vi "Create ActorRef Queue.vi"(11 "Core In":refnum<class "Core.lvclass">) -> (0 "Error Out":errorcluster, 3 "Core Out":refnum<class "Core.lvclass">)   [LabVIEW 2019, in "Core.lvlib" / "Core.lvclass"]
uses:
  Core.lvclass
  C:/Projekty/_Wewnetrzne/PC_ActorFramework/07_Program/LABVIEW/02_Source/Modules/ModuleAbstract/ModuleAbstract.lvclass
  Containers/ActorRefContainer/ActorRefContainer.lvclass
  Containers/ActorRefContainer/ActorRefContainer.lvclass/ActorRefContainer.ctl
  Core.lvclass/Core.ctl
  ModuleAbstract/ModuleAbstract.lvclass/ModuleAbstract.ctl
  <vilib>/ActorFramework/Message Enqueuer/Message Enqueuer.lvclass
  ModuleAbstract/ModuleAbstract.lvclass
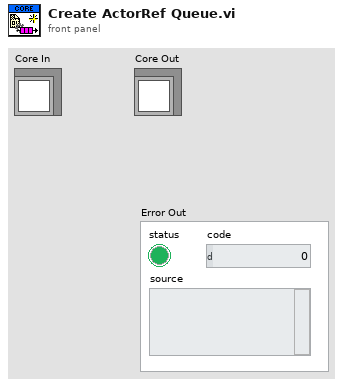
[diagram p1: front panel]
types:
  T1 = cluster{"Core":cluster{"ModRef":refnum<class "Message Enqueuer.lvclass">, "UIRef":refnum<class "Message Enqueuer.lvclass">}}
  T2 = cluster{"EventLog":cluster{"ModRef":refnum<class "Message Enqueuer.lvclass">, "UIRef":refnum<class "Message Enqueuer.lvclass">}}
  T3 = cluster{"ModRef":refnum<class "Message Enqueuer.lvclass">, "UIRef":refnum<class "Message Enqueuer.lvclass">}[]
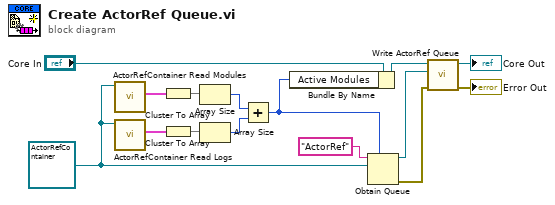
[diagram p0: block diagram]
diagram:
  w9 = refnum<class "ActorRefContainer.lvclass"> refnum ("ActorRefContainer.lvlib:ActorRefContainer.lvclass")
  n1 = call "ActorRefContainer Read Modules.vi"("ActorRefContainer in"=w9) -> ("Modules"=w8:T1)  [unwired: 8 in, 2 out]
  n2 = call "ActorRefContainer Read Logs.vi"("ActorRefContainer in"=w9) -> ("Logs"=w6:T2)  [unwired: 8 in, 2 out]
  n3 = Cluster To Array(cluster=w8) -> (array=w14:T3)
  n4 = Cluster To Array(cluster=w6) -> (array=w7:T3)
  n5 = Array Size(array=w14) -> (size(s)=w4:i32)
  n6 = Array Size(array=w7) -> (size(s)=w5:i32)
  n7 = Add(x=w4, y=w5) -> (x+y=w2:i32)
  n8 = Bundle By Name(cluster="Core In", "Active Modules"=w2) -> (w3:refnum<class "Core.lvclass">)
  n9 = Obtain Queue(max queue size (-1, unlimited)=w2, name (unnamed)="ActorRef", element data type=w9) -> (queue out=w1:refnum<queue>, error out=w11:errorcluster)  [unwired: 2 in, 1 out]
  n10 = call "Write ActorRef Queue.vi"("error in (no error)"=w11, "ActorRef Queue"=w1, "ModuleAbstract in"=w3) -> ("error out"=→"Error Out":errorcluster, "ModuleAbstract out"=→"Core Out":refnum<class "Core.lvclass">)  [unwired: 7 in]
